vi "Write.vi"(0 "Sift Client in":refnum<class "Sift Client.lvclass">, 5 "Values":variant[](array[variant]), 7 "Timestamp":T2, 9 "Flow Name":string="default_flow_name", 11 "error in (no error)":errorcluster) -> (4 "Sift Client out":refnum<class "Sift Client.lvclass">, 15 "error out":errorcluster)   [LabVIEW 2024, in "Sift Client.lvlib" / "Sift Client.lvclass"]
doc: "Write a batch of values for a single flow.\n\nIMPORTANT: The order of data in Values MUST be the same as the order channels were registered for the specified flow.\n\nValues is an array values of the different channels in the specified flow. Since each channel can be a different data type, an array of Variants shall be used. \n\nIf no Flow Name is provided the default will be used."
uses:
  Sift Client.lvclass
  Private/Typedefs/Ingestion/Timestamp.ctl
  Private/Typedefs/Ingestion/Sample.ctl
  Sift Client.lvclass/Sift Client.ctl
  <vilib>/Utility/error.llb/Error Cluster From Error Code.vi
  <vilib>/ErrorRing/Error Ring.xnode
  <userlib>/_OpenG.lib/error/error.llb/openg_error.lvlib
  Sift Client.lvlib
panel:
  in  "Sample":T1
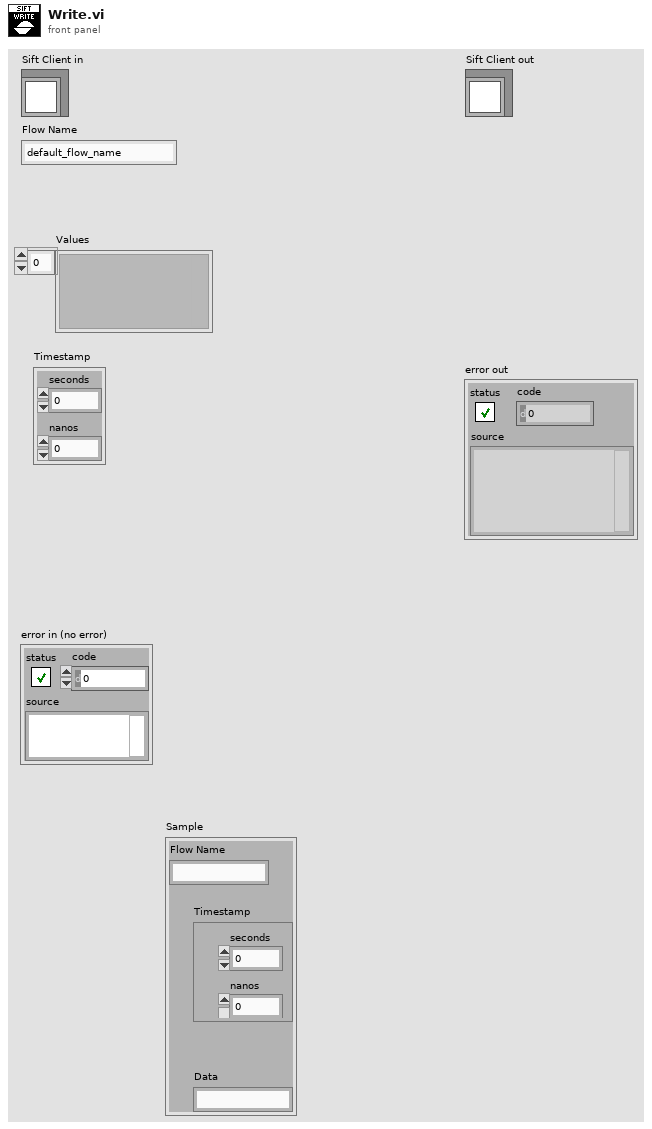
[diagram p1: front panel]
types:
  T1 = typedef "Sift Client.lvlib/Sample.ctl" = cluster{"Flow Name":string, "Timestamp":T2, "Data":string}
  T2 = typedef "Sift Client.lvlib/Timestamp.ctl" = cluster{"seconds":i64, "nanos":i32}
  T3 = typedef "Sift Client.lvlib/Flow Config.ctl" = cluster{"name":string, "channels":T4[]}
  T4 = typedef "Sift Client.lvlib/Channel Config.ctl" = cluster{"name":string, "data_type":T5, "description":string, "component":string, "unit":string, "bit_field_elements":T6[], "enum_types":T7[]}
  T5 = typedef "Sift Client.lvlib/Data Type.ctl" = enum8{"double", "float", "uint64", "int64", "uint32", "int32", "bool", "bit field", "enum"}
  T6 = typedef "Sift Client.lvlib/Bit Field.ctl" = cluster{"index":u32, "bit_count":u32, "name":string}
  T7 = typedef "Sift Client.lvlib/Enum.ctl" = cluster{"Key":u32, "Name":string}
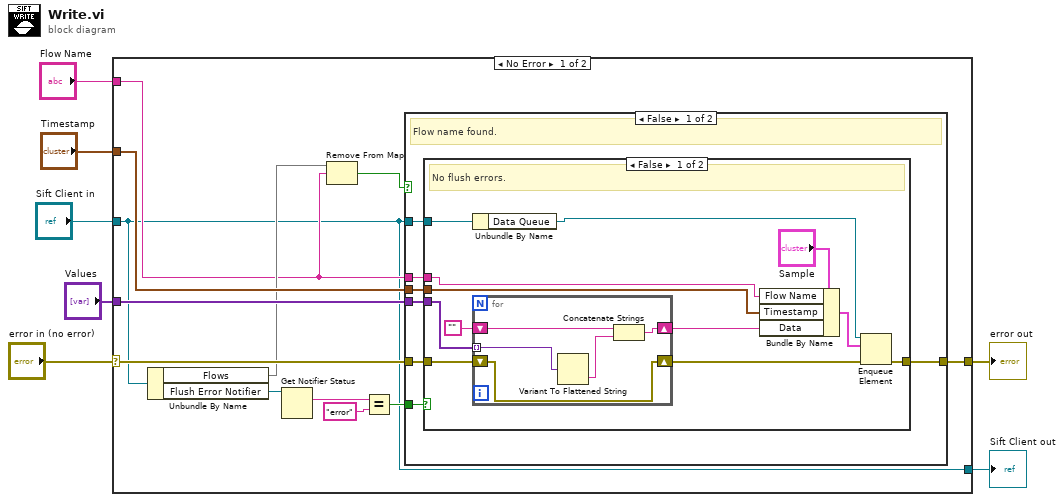
[diagram p0: block diagram]
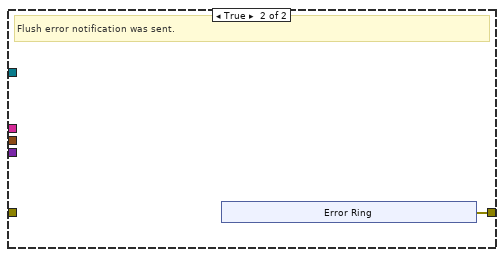
[diagram p2: hidden frame]
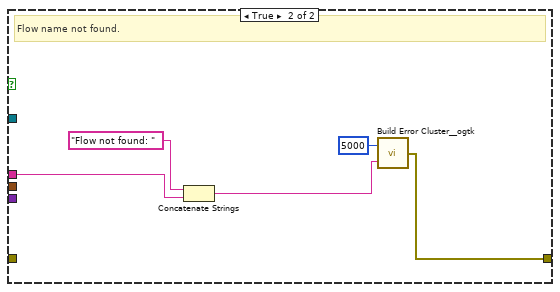
[diagram p3: hidden frame]
diagram:
  n1 = case shown="No Error" "error in (no error)" {
    selector: "error in (no error)" -> [w19 w56]
    tunnel: [w17 w56] -> w6
    tunnel: [w8 w55] -> w4
    tunnel: "Sift Client in" -> [w8 w55]
    tunnel: "Values" -> [w16 _]
    tunnel: "Timestamp" -> [w18 _]
    tunnel: "Flow Name" -> [w14 _]
    frame No Error {
      n2 = Unbundle By Name(w8) -> ("Flows"=w15:map{string, T3}, "Flush Error Notifier"=w13:refnum<notifier>)
      n3 = Get Notifier Status(notifier=w13) -> (current notification=w12:string)  [unwired: 1 in, 4 out]
      n4 = Remove From Map(10:w14, 11:w15) -> (2:w10:bool)  [unwired: 2 out]
      n5 = Equal?(x=w12, y="error") -> (x = y?=w9:bool)
      n6 = case shown="False" w10 {
        tunnel: w19 -> [w26 _]
        tunnel: w18 -> [w25 _]
        tunnel: [w24 w50] -> w17
        tunnel: w16 -> [w23 _]
        tunnel: w14 -> [w22 w52]
        tunnel: w8 -> [w21 _]
        tunnel: w9 -> [w20 _]
        frame False {
          # "Flow name found."
          n7 = case shown="False" w20 {
            tunnel: w26 -> [w34 _]
            tunnel: w21 -> [w31 _]
            tunnel: w25 -> [w37 _]
            tunnel: [w27 w44] -> w24
            tunnel: w23 -> [w35 _]
            tunnel: w22 -> [w36 _]
            frame False {
              # "No flush errors."
              n8 = Unbundle By Name(w31) -> ("Data Queue"=w30:refnum<queue>)
              n9 = for {
                tunnel: w35 -> [w41] mode=indexing
                shift-right: [w43] -> w33
                shift-left: "" -> [w42]
                shift-right: [w39] -> w28
                shift-left: w34 -> [w39]
                n10 = Variant To Flattened String(Variant=w41) -> (data string=w40:string)  [unwired: 1 out]
                n11 = Concatenate Strings(w42, w40) -> (w43:string)
              }
              n12 = Bundle By Name(cluster="Sample", "Flow Name"=w36, "Timestamp"=w37, "Data"=w33) -> (w29:T1)
              n13 = Enqueue Element(queue=w30, element=w29, error in (no error)=w28) -> (error out=w27:errorcluster)  [unwired: 1 in, 2 out]
            }
            frame True {
              # "Flush error notification was sent."
              n14 = xnode "Error Ring"() -> ("error out"=w44:errorcluster)
            }
          }
        }
        frame True {
          # "Flow name not found."
          n15 = Concatenate Strings("Flow not found: ", w52) -> (w51:string)
          n16 = call <userlib>:"Build Error Cluster__ogtk.vi"("String to Prepend to source (\"\")"=w51, "code"=5000) -> ("error out"=w50:errorcluster)
        }
      }
    }
    frame Error {
    }
  }
  "error out" <- w6
  "Sift Client out" <- w4
